vi "Obtain UART.vi"(4 "RX GPIO":T1=17, 5 "Purpose (\"UART\")":string="UART", 6 "TX GPIO":T1=16, 7 "UART #":T2, 8 "error in (no error)":errorcluster, 9 "Term Char (None)":string, 10 "Baud":u32=115200, 11 "Session in":refnum<class "Session.lvclass">) -> (0 "error out":errorcluster, 2 "UART":refnum<class "UART.lvclass">, 3 "Session out":refnum<class "Session.lvclass">)   [LabVIEW 2020, in "CTI.lvlib" / "Session.lvclass"]
uses:
  Session.lvclass
  UART Number.ctl
  GPIO Number.ctl
  UART/UART.lvclass
  UART Pins.ctl
  Session.lvclass/Session.ctl
  5d41f6f2-78eb-42d5-8031-5b57c1ee8460.vi
  5d41f6f2-78eb-42d5-8031-5b57c1ee8460.vi/1ebac61a-bcc0-4be5-9ea8-8faf7576f3c5.vi
  Is Full Errors.vi
  Check Errors.vi
  CTI.lvlib
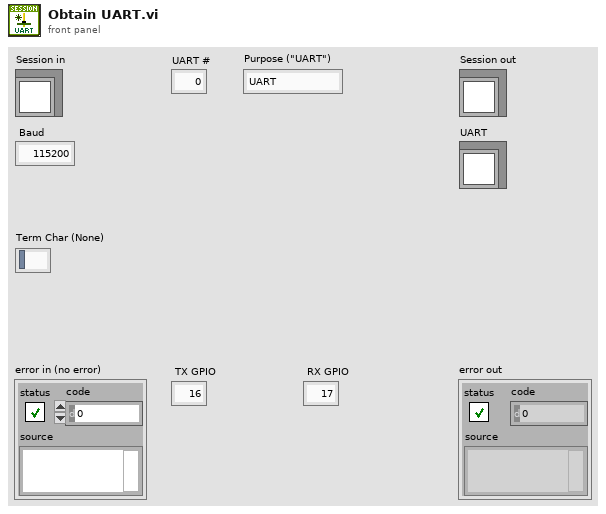
[diagram p1: front panel]
types:
  T1 = typedef "CTI.lvlib/GPIO Number.ctl" = i8
  T2 = typedef "CTI.lvlib/UART Number.ctl" = i8
  T3 = typedef "CTI.lvlib/UART Pins.ctl" = cluster{"TX GPIO":T1, "RX GPIO":T1}
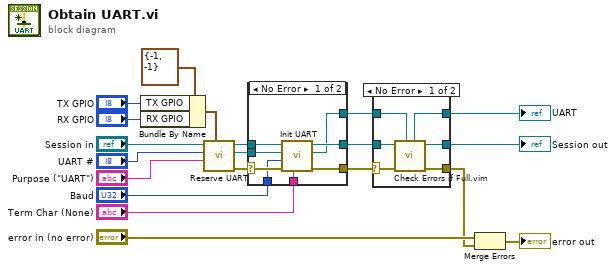
[diagram p0: block diagram]
diagram:
  n1 = Bundle By Name(cluster=T3 {"TX GPIO"=-1, "RX GPIO"=-1} ("UART Pins"), "TX GPIO"="TX GPIO", "RX GPIO"="RX GPIO") -> (w17:T3)
  n2 = call "Reserve UART.vi"("UART Pins"=w17, "Purpose"="Purpose (\"UART\")", "UART #"="UART #", "Session in"="Session in") -> ("error out"=w12:errorcluster, "UART"=w10:refnum<class "UART.lvclass">, "Session out"=w11:refnum<class "Session.lvclass">)  [unwired: 5 in]
  n3 = case shown="No Error" w12 {
    selector: w12 -> [w26 w29]
    tunnel: w11 -> [w28 w30]
    tunnel: w10 -> [w27 _]
    tunnel: "Baud" -> [w25 _]
    tunnel: "Term Char (None)" -> [w24 _]
    tunnel: [w23 w30] -> w6
    tunnel: [w22 w29] -> w7
    tunnel: [w21 _] -> w5
    frame No Error {
      n4 = call-dynamic "Init UART.vi"("Term Char"=w24, "error in (no error)"=w26, "Baud"=w25, "UART In"=w27, "Session in"=w28) -> ("error out"=w22:errorcluster, "UART"=w21:refnum<class "UART.lvclass">, "Session out"=w23:refnum<class "Session.lvclass">)  [unwired: 4 in]
    }
    frame Error {
    }
  }
  n5 = case shown="No Error" w7 {
    selector: w7 -> [w35 w37]
    tunnel: w6 -> [w36 w38]
    tunnel: w5 -> [w34 _]
    tunnel: [w33 _] -> w4
    tunnel: [w32 w38] -> w3
    tunnel: [w31 w37] -> w1
    frame No Error {
      n6 = call "Check Errors if Full.vim"("Resource In"=w34, "error in (no error)"=w35, "Session in"=w36) -> ("error out"=w31:errorcluster, "Session out"=w32:refnum<class "Session.lvclass">, "Resource"=w33:refnum<class "UART.lvclass">)  [unwired: 6 in]
    }
    frame Error {
    }
  }
  "Session out" <- w3
  "UART" <- w4
  n7 = Merge Errors("error in (no error)", w1) -> (→"error out":errorcluster)
